vi "例4-29（1）.vi"() -> ()   [LabVIEW 2019]
panel:
  in  "停止":bool
  out "波形图表":T1(graph)
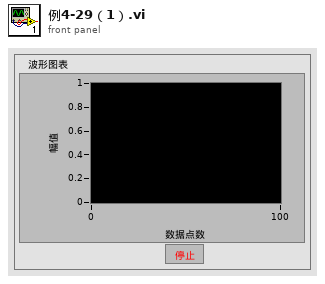
[diagram p1: front panel]
types:
  T1 = cluster{"number: 0 to 1":dbl, "number: 0 to 1":dbl}
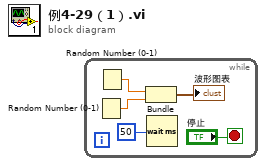
[diagram p0: block diagram]
diagram:
  n1 = while {
    stop <- "停止" stop-if-true
    n2 = Random Number (0-1)() -> (number: 0 to 1=w5:dbl)
    n3 = Random Number (0-1)() -> (number: 0 to 1=w4:dbl)
    n4 = Bundle("number: 0 to 1"=w4, "number: 0 to 1"=w5) -> (→"波形图表":T1)  [unwired: 1 in]
    n5 = Wait (ms)(milliseconds to wait=50) -> ()  [unwired: 1 out]
  }
